vi "Parse.vi"(8 "Error In":errorcluster, 11 "object in":refnum<class "2024_13.lvclass">) -> (0 "Error Out":errorcluster, 3 "object out":refnum<class "2024_13.lvclass">)   [LabVIEW 2023, in "2024_13.lvclass"]
uses:
  2024_13.lvclass
  Game.ctl
  Common/AOC_XY.ctl
  2024_13.lvclass/2024_13.ctl
  <vilib>/Utility/error.llb/Trim Whitespace One-Sided.vi
  <userlib>/_OpenG.lib/string/string.llb/openg_string.lvlib
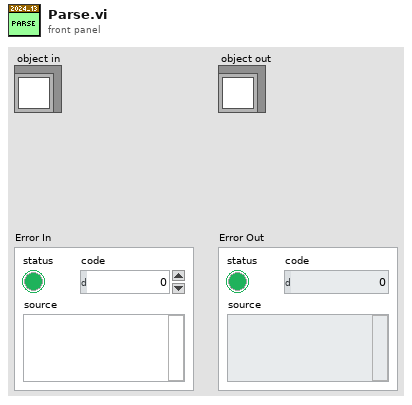
[diagram p1: front panel]
types:
  T1 = typedef "2024_13.lvclass/Game.ctl" = cluster{"A":T2, "B":T2, "Prize":T2}
  T2 = typedef "AOC_XY.ctl" = cluster{"X":u64, "Y":u64}
diagram:
  (unwired) "Button A: X+94, Y+34\nButton B: X+22, Y+67\nPrize: X=8400, Y=5400\n\nButton A: X+26, Y+66\nButton B: X+67, Y+21\nPrize: X=12748, Y=12176\n\nButton A: X+17, Y+86\nButton B: X+84, Y+37\nPrize: X=7870, Y=6450\n\nButton A: X+69, Y+23\nButton B: X+27, Y+71\nPrize: X=18641, Y=10279" ("PuzzleInput")
  n1 = call <vilib>:"Trim Whitespace.vi"("string"="Button A: X+97, Y+12\nButton B: X+52, Y+63\nPrize: X=10471, Y=4350\n\nButton A: X+79, Y+41\nButton B: X+29, Y+68\nPrize: X=7216, Y=8987\n\nButton A: X+13, Y+68\nButton B: X+46, Y+16\nPrize: X=1226, Y=8336\n\nButton A: X+14, Y+42\nButton B: X+63, Y+23\nPrize: X=15649, Y=1769\n\nButton A: X+59, Y+19\nButton B: X+53, Y+95\nPrize: X=8976, Y=10450\n\nButton A: X+91, Y+84\nButton B: X+19, Y+92\nPrize: X=9023, Y=13020\n\nButton A: X+14, Y+33\nButton B: X+26, Y+12\nPrize: X=4032, Y=8054\n\nButton A: X+69, Y+83\nButton B: X+70, Y+18\nPrize: X=8868, Y=8284\n\nButton A: X+14, Y+47\nButton B: X+83, Y+51\nPrize: X=7081, Y=7154\n\nButton A: X+33, Y+67\nButton B: X+50, Y+17\nPrize: X=12916, Y=4279\n\nButton A: X+22, Y+75\nButton B: X+77, Y+23\nPrize: X=12981, Y=9742\n\nButton A: X+90, Y+30\nButton B: X+17, Y+33\nPrize: X=6270, Y=2910\n\nButton A: X+62, Y+11\nButton B: X+43, Y+65\nPrize: X=3850, Y=1601\n\nButton A: X+48, Y+21\nButton B: X+21, Y+33\nPrize: X=8108, Y=1334\n\nButton A: X+12, Y+40\nButton B: X+49, Y+23\nPrize: X=12471, Y=11957\n\nButton A: X+86, Y+11\nButton B: X+56, Y+69\nPrize: X=4404, Y=1058\n\nButton A: X+80, Y+26\nButton B: X+11, Y+57\nPrize: X=6899, Y=5923\n\nButton A: X+25, Y+51\nButton B: X+59, Y+24\nPrize: X=14076, Y=10916\n\nButton A: X+48, Y+46\nButton B: X+13, Y+94\nPrize: X=1915, Y=6320\n\nButton A: X+47, Y+32\nButton B: X+20, Y+44\nPrize: X=19516, Y=14572\n\nButton A: X+84, Y+21\nButton B: X+13, Y+89\nPrize: X=4350, Y=2631\n\nButton A: X+29, Y+85\nButton B: X+33, Y+26\nPrize: X=4361, Y=7973\n\nButton A: X+78, Y+35\nButton B: X+11, Y+42\nPrize: X=9808, Y=10623\n\nButton A: X+35, Y+64\nButton B: X+38, Y+15\nPrize: X=4993, Y=274\n\nButton A: X+18, Y+47\nButton B: X+54, Y+15\nPrize: X=10646, Y=16999\n\nButton A: X+99, Y+55\nButton B: X+18, Y+75\nPrize: X=5256, Y=5455\n\nButton A: X+83, Y+91\nButton B: X+11, Y+58\nPrize: X=3635, Y=4261\n\nButton A: X+60, Y+27\nButton B: X+29, Y+56\nPrize: X=740, Y=11114\n\nButton A: X+59, Y+15\nButton B: X+29, Y+75\nPrize: X=14539, Y=13025\n\nButton A: X+67, Y+23\nButton B: X+11, Y+57\nPrize: X=2430, Y=2218\n\nButton A: X+80, Y+45\nButton B: X+37, Y+82\nPrize: X=9822, Y=10787\n\nButton A: X+11, Y+45\nButton B: X+51, Y+23\nPrize: X=1269, Y=18697\n\nButton A: X+56, Y+32\nButton B: X+16, Y+50\nPrize: X=9080, Y=15276\n\nButton A: X+93, Y+93\nButton B: X+11, Y+90\nPrize: X=4103, Y=11529\n\nButton A: X+24, Y+21\nButton B: X+12, Y+51\nPrize: X=2016, Y=3627\n\nButton A: X+72, Y+41\nButton B: X+25, Y+80\nPrize: X=3812, Y=3486\n\nButton A: X+29, Y+14\nButton B: X+22, Y+53\nPrize: X=2677, Y=14205\n\nButton A: X+56, Y+18\nButton B: X+19, Y+69\nPrize: X=4292, Y=8432\n\nButton A: X+64, Y+16\nButton B: X+14, Y+50\nPrize: X=3752, Y=536\n\nButton A: X+45, Y+31\nButton B: X+26, Y+59\nPrize: X=4694, Y=5247\n\nButton A: X+61, Y+21\nButton B: X+19, Y+48\nPrize: X=3931, Y=257\n\nButton A: X+13, Y+36\nButton B: X+68, Y+26\nPrize: X=17218, Y=17896\n\nButton A: X+15, Y+81\nButton B: X+31, Y+21\nPrize: X=2580, Y=7344\n\nButton A: X+78, Y+51\nButton B: X+12, Y+34\nPrize: X=3380, Y=16870\n\nButton A: X+86, Y+29\nButton B: X+52, Y+60\nPrize: X=5118, Y=2745\n\nButton A: X+12, Y+49\nButton B: X+77, Y+16\nPrize: X=7847, Y=7211\n\nButton A: X+30, Y+49\nButton B: X+48, Y+19\nPrize: X=1034, Y=15377\n\nButton A: X+25, Y+61\nButton B: X+26, Y+12\nPrize: X=6825, Y=14177\n\nButton A: X+59, Y+20\nButton B: X+11, Y+23\nPrize: X=13324, Y=946\n\nButton A: X+36, Y+54\nButton B: X+29, Y+13\nPrize: X=4435, Y=12219\n\nButton A: X+17, Y+77\nButton B: X+61, Y+17\nPrize: X=2681, Y=5661\n\nButton A: X+41, Y+19\nButton B: X+25, Y+55\nPrize: X=4484, Y=9416\n\nButton A: X+26, Y+68\nButton B: X+70, Y+26\nPrize: X=8284, Y=10434\n\nButton A: X+54, Y+11\nButton B: X+25, Y+78\nPrize: X=11040, Y=7758\n\nButton A: X+85, Y+23\nButton B: X+54, Y+74\nPrize: X=2400, Y=2728\n\nButton A: X+93, Y+29\nButton B: X+13, Y+22\nPrize: X=7293, Y=2328\n\nButton A: X+23, Y+87\nButton B: X+48, Y+20\nPrize: X=2279, Y=4743\n\nButton A: X+83, Y+34\nButton B: X+32, Y+43\nPrize: X=7734, Y=4035\n\nButton A: X+25, Y+61\nButton B: X+83, Y+44\nPrize: X=6884, Y=5225\n\nButton A: X+27, Y+58\nButton B: X+98, Y+47\nPrize: X=7921, Y=3934\n\nButton A: X+31, Y+57\nButton B: X+33, Y+14\nPrize: X=3052, Y=3838\n\nButton A: X+96, Y+18\nButton B: X+77, Y+97\nPrize: X=6503, Y=6751\n\nButton A: X+11, Y+29\nButton B: X+71, Y+36\nPrize: X=1000, Y=671\n\nButton A: X+25, Y+53\nButton B: X+44, Y+20\nPrize: X=13129, Y=17325\n\nButton A: X+33, Y+13\nButton B: X+50, Y+66\nPrize: X=3194, Y=9314\n\nButton A: X+54, Y+15\nButton B: X+24, Y+64\nPrize: X=19418, Y=8601\n\nButton A: X+13, Y+46\nButton B: X+56, Y+14\nPrize: X=10671, Y=11208\n\nButton A: X+35, Y+91\nButton B: X+25, Y+14\nPrize: X=2700, Y=6153\n\nButton A: X+85, Y+25\nButton B: X+16, Y+97\nPrize: X=2407, Y=1354\n\nButton A: X+24, Y+12\nButton B: X+13, Y+30\nPrize: X=3299, Y=3318\n\nButton A: X+17, Y+46\nButton B: X+50, Y+24\nPrize: X=17242, Y=6760\n\nButton A: X+20, Y+43\nButton B: X+26, Y+14\nPrize: X=2474, Y=748\n\nButton A: X+19, Y+78\nButton B: X+90, Y+12\nPrize: X=9966, Y=7668\n\nButton A: X+96, Y+77\nButton B: X+26, Y+73\nPrize: X=3708, Y=5790\n\nButton A: X+37, Y+77\nButton B: X+51, Y+15\nPrize: X=13364, Y=12440\n\nButton A: X+30, Y+78\nButton B: X+76, Y+31\nPrize: X=6378, Y=3588\n\nButton A: X+60, Y+26\nButton B: X+13, Y+25\nPrize: X=10780, Y=7426\n\nButton A: X+33, Y+40\nButton B: X+59, Y+16\nPrize: X=4212, Y=3440\n\nButton A: X+30, Y+11\nButton B: X+25, Y+40\nPrize: X=1145, Y=1499\n\nButton A: X+14, Y+30\nButton B: X+48, Y+15\nPrize: X=4416, Y=3840\n\nButton A: X+45, Y+68\nButton B: X+59, Y+25\nPrize: X=6633, Y=5404\n\nButton A: X+34, Y+62\nButton B: X+44, Y+19\nPrize: X=9234, Y=16930\n\nButton A: X+65, Y+12\nButton B: X+16, Y+42\nPrize: X=13586, Y=10016\n\nButton A: X+16, Y+86\nButton B: X+63, Y+54\nPrize: X=2515, Y=5264\n\nButton A: X+40, Y+88\nButton B: X+91, Y+56\nPrize: X=3728, Y=7048\n\nButton A: X+43, Y+79\nButton B: X+91, Y+30\nPrize: X=5407, Y=1977\n\nButton A: X+87, Y+16\nButton B: X+86, Y+76\nPrize: X=3366, Y=2244\n\nButton A: X+39, Y+74\nButton B: X+94, Y+32\nPrize: X=6130, Y=6216\n\nButton A: X+91, Y+50\nButton B: X+24, Y+71\nPrize: X=9174, Y=7411\n\nButton A: X+81, Y+55\nButton B: X+14, Y+95\nPrize: X=4359, Y=7320\n\nButton A: X+26, Y+78\nButton B: X+79, Y+58\nPrize: X=8792, Y=11698\n\nButton A: X+81, Y+58\nButton B: X+21, Y+70\nPrize: X=8145, Y=9130\n\nButton A: X+29, Y+60\nButton B: X+83, Y+29\nPrize: X=9583, Y=6839\n\nButton A: X+72, Y+27\nButton B: X+23, Y+63\nPrize: X=16485, Y=8540\n\nButton A: X+18, Y+30\nButton B: X+47, Y+13\nPrize: X=3031, Y=8157\n\nButton A: X+36, Y+14\nButton B: X+52, Y+70\nPrize: X=19584, Y=5184\n\nButton A: X+13, Y+36\nButton B: X+32, Y+23\nPrize: X=12901, Y=6580\n\nButton A: X+34, Y+66\nButton B: X+57, Y+24\nPrize: X=13320, Y=4832\n\nButton A: X+79, Y+26\nButton B: X+65, Y+85\nPrize: X=7528, Y=2732\n\nButton A: X+20, Y+58\nButton B: X+96, Y+75\nPrize: X=3288, Y=5874\n\nButton A: X+89, Y+24\nButton B: X+35, Y+67\nPrize: X=3458, Y=5595\n\nButton A: X+63, Y+81\nButton B: X+67, Y+22\nPrize: X=4988, Y=3206\n\nButton A: X+17, Y+55\nButton B: X+54, Y+13\nPrize: X=17532, Y=19258\n\nButton A: X+30, Y+94\nButton B: X+93, Y+32\nPrize: X=2874, Y=4336\n\nButton A: X+31, Y+17\nButton B: X+24, Y+40\nPrize: X=2311, Y=8105\n\nButton A: X+58, Y+27\nButton B: X+19, Y+60\nPrize: X=6022, Y=6398\n\nButton A: X+13, Y+67\nButton B: X+84, Y+29\nPrize: X=2843, Y=2323\n\nButton A: X+56, Y+12\nButton B: X+23, Y+81\nPrize: X=2380, Y=11120\n\nButton A: X+15, Y+65\nButton B: X+56, Y+24\nPrize: X=5230, Y=5170\n\nButton A: X+19, Y+47\nButton B: X+72, Y+34\nPrize: X=17967, Y=11841\n\nButton A: X+16, Y+41\nButton B: X+78, Y+60\nPrize: X=5144, Y=4789\n\nButton A: X+52, Y+15\nButton B: X+16, Y+65\nPrize: X=19732, Y=7355\n\nButton A: X+21, Y+81\nButton B: X+71, Y+16\nPrize: X=17221, Y=9366\n\nButton A: X+61, Y+33\nButton B: X+49, Y+87\nPrize: X=8507, Y=9381\n\nButton A: X+67, Y+21\nButton B: X+15, Y+52\nPrize: X=16737, Y=7411\n\nButton A: X+33, Y+49\nButton B: X+34, Y+11\nPrize: X=6660, Y=4300\n\nButton A: X+19, Y+81\nButton B: X+96, Y+33\nPrize: X=10734, Y=10392\n\nButton A: X+60, Y+13\nButton B: X+63, Y+65\nPrize: X=7395, Y=3913\n\nButton A: X+15, Y+21\nButton B: X+96, Y+35\nPrize: X=6417, Y=3815\n\nButton A: X+20, Y+39\nButton B: X+57, Y+27\nPrize: X=611, Y=4760\n\nButton A: X+68, Y+97\nButton B: X+87, Y+37\nPrize: X=11894, Y=9824\n\nButton A: X+13, Y+81\nButton B: X+59, Y+12\nPrize: X=18946, Y=3392\n\nButton A: X+30, Y+83\nButton B: X+57, Y+11\nPrize: X=3482, Y=19301\n\nButton A: X+94, Y+11\nButton B: X+35, Y+92\nPrize: X=11544, Y=7680\n\nButton A: X+45, Y+19\nButton B: X+30, Y+45\nPrize: X=11315, Y=17659\n\nButton A: X+25, Y+42\nButton B: X+79, Y+21\nPrize: X=7695, Y=3990\n\nButton A: X+95, Y+91\nButton B: X+55, Y+13\nPrize: X=10575, Y=9217\n\nButton A: X+27, Y+46\nButton B: X+81, Y+26\nPrize: X=5508, Y=2776\n\nButton A: X+20, Y+53\nButton B: X+29, Y+17\nPrize: X=10985, Y=16700\n\nButton A: X+55, Y+74\nButton B: X+58, Y+20\nPrize: X=8888, Y=8128\n\nButton A: X+40, Y+27\nButton B: X+19, Y+43\nPrize: X=5535, Y=1095\n\nButton A: X+19, Y+72\nButton B: X+54, Y+22\nPrize: X=3261, Y=2678\n\nButton A: X+79, Y+39\nButton B: X+38, Y+75\nPrize: X=7120, Y=6102\n\nButton A: X+26, Y+91\nButton B: X+99, Y+25\nPrize: X=1223, Y=2673\n\nButton A: X+15, Y+28\nButton B: X+58, Y+23\nPrize: X=1519, Y=5600\n\nButton A: X+18, Y+53\nButton B: X+71, Y+27\nPrize: X=11055, Y=3487\n\nButton A: X+14, Y+50\nButton B: X+52, Y+18\nPrize: X=3908, Y=8576\n\nButton A: X+38, Y+17\nButton B: X+23, Y+50\nPrize: X=7788, Y=8394\n\nButton A: X+72, Y+20\nButton B: X+19, Y+68\nPrize: X=10586, Y=4272\n\nButton A: X+28, Y+66\nButton B: X+62, Y+12\nPrize: X=19418, Y=7934\n\nButton A: X+11, Y+20\nButton B: X+49, Y+24\nPrize: X=2957, Y=2252\n\nButton A: X+60, Y+11\nButton B: X+27, Y+84\nPrize: X=3146, Y=1936\n\nButton A: X+18, Y+11\nButton B: X+11, Y+41\nPrize: X=9360, Y=18112\n\nButton A: X+70, Y+31\nButton B: X+15, Y+62\nPrize: X=13135, Y=7958\n\nButton A: X+74, Y+35\nButton B: X+11, Y+41\nPrize: X=19668, Y=14478\n\nButton A: X+53, Y+89\nButton B: X+54, Y+23\nPrize: X=9521, Y=10100\n\nButton A: X+13, Y+61\nButton B: X+68, Y+28\nPrize: X=11028, Y=12380\n\nButton A: X+42, Y+29\nButton B: X+20, Y+74\nPrize: X=1906, Y=1617\n\nButton A: X+44, Y+13\nButton B: X+23, Y+60\nPrize: X=13690, Y=9554\n\nButton A: X+54, Y+16\nButton B: X+11, Y+23\nPrize: X=3792, Y=4614\n\nButton A: X+28, Y+11\nButton B: X+34, Y+63\nPrize: X=13092, Y=15599\n\nButton A: X+61, Y+14\nButton B: X+33, Y+73\nPrize: X=18520, Y=772\n\nButton A: X+64, Y+29\nButton B: X+14, Y+78\nPrize: X=3988, Y=4530\n\nButton A: X+18, Y+45\nButton B: X+54, Y+26\nPrize: X=18170, Y=10118\n\nButton A: X+70, Y+26\nButton B: X+11, Y+43\nPrize: X=6905, Y=329\n\nButton A: X+72, Y+17\nButton B: X+27, Y+58\nPrize: X=7461, Y=6253\n\nButton A: X+57, Y+45\nButton B: X+18, Y+85\nPrize: X=2340, Y=5670\n\nButton A: X+17, Y+81\nButton B: X+47, Y+35\nPrize: X=5532, Y=8220\n\nButton A: X+14, Y+60\nButton B: X+78, Y+22\nPrize: X=10172, Y=5672\n\nButton A: X+62, Y+13\nButton B: X+17, Y+65\nPrize: X=7711, Y=8089\n\nButton A: X+22, Y+38\nButton B: X+40, Y+21\nPrize: X=15254, Y=15785\n\nButton A: X+83, Y+39\nButton B: X+32, Y+71\nPrize: X=2416, Y=3038\n\nButton A: X+29, Y+62\nButton B: X+68, Y+18\nPrize: X=6454, Y=3990\n\nButton A: X+15, Y+38\nButton B: X+72, Y+33\nPrize: X=3575, Y=8334\n\nButton A: X+81, Y+15\nButton B: X+13, Y+83\nPrize: X=11268, Y=10108\n\nButton A: X+67, Y+17\nButton B: X+12, Y+76\nPrize: X=11957, Y=5399\n\nButton A: X+13, Y+97\nButton B: X+44, Y+54\nPrize: X=2788, Y=7636\n\nButton A: X+14, Y+47\nButton B: X+68, Y+30\nPrize: X=2678, Y=9911\n\nButton A: X+75, Y+16\nButton B: X+22, Y+26\nPrize: X=1049, Y=586\n\nButton A: X+16, Y+77\nButton B: X+38, Y+25\nPrize: X=2368, Y=7607\n\nButton A: X+75, Y+91\nButton B: X+77, Y+20\nPrize: X=4076, Y=3991\n\nButton A: X+64, Y+19\nButton B: X+35, Y+74\nPrize: X=8653, Y=7594\n\nButton A: X+33, Y+81\nButton B: X+57, Y+15\nPrize: X=10661, Y=2849\n\nButton A: X+11, Y+52\nButton B: X+70, Y+22\nPrize: X=1390, Y=2864\n\nButton A: X+21, Y+40\nButton B: X+21, Y+13\nPrize: X=5954, Y=5203\n\nButton A: X+52, Y+21\nButton B: X+13, Y+64\nPrize: X=11131, Y=9958\n\nButton A: X+11, Y+42\nButton B: X+95, Y+52\nPrize: X=1604, Y=4260\n\nButton A: X+63, Y+13\nButton B: X+22, Y+82\nPrize: X=670, Y=17610\n\nButton A: X+16, Y+88\nButton B: X+84, Y+74\nPrize: X=3184, Y=6648\n\nButton A: X+77, Y+14\nButton B: X+92, Y+88\nPrize: X=13208, Y=8816\n\nButton A: X+63, Y+67\nButton B: X+82, Y+13\nPrize: X=8310, Y=3940\n\nButton A: X+57, Y+16\nButton B: X+17, Y+48\nPrize: X=10242, Y=5248\n\nButton A: X+17, Y+72\nButton B: X+36, Y+37\nPrize: X=3710, Y=5667\n\nButton A: X+69, Y+22\nButton B: X+29, Y+54\nPrize: X=5207, Y=5330\n\nButton A: X+23, Y+82\nButton B: X+49, Y+11\nPrize: X=2320, Y=2070\n\nButton A: X+66, Y+27\nButton B: X+16, Y+45\nPrize: X=11344, Y=9314\n\nButton A: X+56, Y+12\nButton B: X+23, Y+66\nPrize: X=13879, Y=14258\n\nButton A: X+60, Y+22\nButton B: X+18, Y+91\nPrize: X=1668, Y=4494\n\nButton A: X+33, Y+11\nButton B: X+31, Y+68\nPrize: X=6069, Y=13315\n\nButton A: X+14, Y+37\nButton B: X+59, Y+14\nPrize: X=2210, Y=5344\n\nButton A: X+80, Y+18\nButton B: X+33, Y+94\nPrize: X=4128, Y=9240\n\nButton A: X+40, Y+17\nButton B: X+28, Y+45\nPrize: X=3436, Y=3526\n\nButton A: X+16, Y+53\nButton B: X+50, Y+22\nPrize: X=642, Y=18961\n\nButton A: X+17, Y+39\nButton B: X+65, Y+23\nPrize: X=9566, Y=11794\n\nButton A: X+66, Y+35\nButton B: X+30, Y+76\nPrize: X=8010, Y=8394\n\nButton A: X+52, Y+75\nButton B: X+37, Y+15\nPrize: X=335, Y=19220\n\nButton A: X+36, Y+29\nButton B: X+30, Y+89\nPrize: X=3690, Y=4334\n\nButton A: X+31, Y+58\nButton B: X+50, Y+20\nPrize: X=8178, Y=17844\n\nButton A: X+82, Y+22\nButton B: X+89, Y+90\nPrize: X=4306, Y=1552\n\nButton A: X+12, Y+42\nButton B: X+99, Y+75\nPrize: X=1173, Y=3291\n\nButton A: X+23, Y+57\nButton B: X+40, Y+19\nPrize: X=2246, Y=9772\n\nButton A: X+18, Y+42\nButton B: X+95, Y+15\nPrize: X=9610, Y=4650\n\nButton A: X+20, Y+57\nButton B: X+59, Y+21\nPrize: X=10072, Y=16868\n\nButton A: X+23, Y+34\nButton B: X+42, Y+15\nPrize: X=6683, Y=16946\n\nButton A: X+55, Y+73\nButton B: X+30, Y+11\nPrize: X=4150, Y=3001\n\nButton A: X+22, Y+82\nButton B: X+73, Y+12\nPrize: X=16713, Y=15870\n\nButton A: X+14, Y+53\nButton B: X+65, Y+35\nPrize: X=3017, Y=4034\n\nButton A: X+25, Y+53\nButton B: X+46, Y+19\nPrize: X=13804, Y=8575\n\nButton A: X+29, Y+13\nButton B: X+38, Y+60\nPrize: X=14048, Y=11678\n\nButton A: X+57, Y+21\nButton B: X+61, Y+83\nPrize: X=6297, Y=7041\n\nButton A: X+18, Y+99\nButton B: X+77, Y+75\nPrize: X=2549, Y=3216\n\nButton A: X+59, Y+22\nButton B: X+17, Y+33\nPrize: X=11044, Y=13465\n\nButton A: X+40, Y+17\nButton B: X+47, Y+77\nPrize: X=17101, Y=14482\n\nButton A: X+34, Y+14\nButton B: X+20, Y+38\nPrize: X=594, Y=572\n\nButton A: X+26, Y+62\nButton B: X+35, Y+11\nPrize: X=6771, Y=8811\n\nButton A: X+20, Y+33\nButton B: X+93, Y+21\nPrize: X=5259, Y=2982\n\nButton A: X+89, Y+60\nButton B: X+13, Y+91\nPrize: X=9182, Y=14167\n\nButton A: X+28, Y+98\nButton B: X+98, Y+63\nPrize: X=5712, Y=8792\n\nButton A: X+67, Y+94\nButton B: X+39, Y+15\nPrize: X=7520, Y=7532\n\nButton A: X+38, Y+17\nButton B: X+25, Y+38\nPrize: X=19009, Y=14132\n\nButton A: X+18, Y+51\nButton B: X+85, Y+39\nPrize: X=9247, Y=7833\n\nButton A: X+40, Y+92\nButton B: X+55, Y+23\nPrize: X=2390, Y=1978\n\nButton A: X+63, Y+39\nButton B: X+24, Y+51\nPrize: X=7448, Y=17612\n\nButton A: X+95, Y+25\nButton B: X+33, Y+64\nPrize: X=11557, Y=8241\n\nButton A: X+40, Y+23\nButton B: X+21, Y+73\nPrize: X=3186, Y=5853\n\nButton A: X+89, Y+81\nButton B: X+13, Y+91\nPrize: X=5270, Y=6538\n\nButton A: X+69, Y+17\nButton B: X+21, Y+64\nPrize: X=10955, Y=8181\n\nButton A: X+59, Y+15\nButton B: X+21, Y+77\nPrize: X=6203, Y=4791\n\nButton A: X+25, Y+45\nButton B: X+36, Y+21\nPrize: X=12604, Y=18854\n\nButton A: X+67, Y+17\nButton B: X+21, Y+70\nPrize: X=7506, Y=17163\n\nButton A: X+78, Y+53\nButton B: X+27, Y+89\nPrize: X=2391, Y=7065\n\nButton A: X+68, Y+26\nButton B: X+23, Y+62\nPrize: X=13179, Y=7794\n\nButton A: X+18, Y+44\nButton B: X+54, Y+16\nPrize: X=18710, Y=4780\n\nButton A: X+16, Y+36\nButton B: X+69, Y+48\nPrize: X=6028, Y=5412\n\nButton A: X+45, Y+24\nButton B: X+34, Y+73\nPrize: X=4185, Y=4701\n\nButton A: X+12, Y+26\nButton B: X+64, Y+29\nPrize: X=8628, Y=3714\n\nButton A: X+53, Y+16\nButton B: X+26, Y+65\nPrize: X=15387, Y=3502\n\nButton A: X+48, Y+17\nButton B: X+49, Y+80\nPrize: X=19364, Y=6034\n\nButton A: X+34, Y+70\nButton B: X+45, Y+21\nPrize: X=3861, Y=2289\n\nButton A: X+39, Y+76\nButton B: X+80, Y+14\nPrize: X=8169, Y=3574\n\nButton A: X+79, Y+35\nButton B: X+45, Y+74\nPrize: X=7247, Y=6887\n\nButton A: X+33, Y+19\nButton B: X+12, Y+49\nPrize: X=7163, Y=16959\n\nButton A: X+24, Y+11\nButton B: X+30, Y+49\nPrize: X=11852, Y=4499\n\nButton A: X+32, Y+11\nButton B: X+25, Y+70\nPrize: X=5331, Y=15303\n\nButton A: X+98, Y+63\nButton B: X+18, Y+68\nPrize: X=5564, Y=5044\n\nButton A: X+85, Y+11\nButton B: X+41, Y+76\nPrize: X=10558, Y=6527\n\nButton A: X+20, Y+48\nButton B: X+45, Y+11\nPrize: X=10755, Y=17297\n\nButton A: X+37, Y+23\nButton B: X+23, Y+51\nPrize: X=12782, Y=14840\n\nButton A: X+37, Y+69\nButton B: X+44, Y+11\nPrize: X=4057, Y=15396\n\nButton A: X+21, Y+43\nButton B: X+55, Y+30\nPrize: X=6148, Y=18269\n\nButton A: X+32, Y+63\nButton B: X+32, Y+17\nPrize: X=8032, Y=16179\n\nButton A: X+81, Y+68\nButton B: X+18, Y+51\nPrize: X=3429, Y=6001\n\nButton A: X+90, Y+27\nButton B: X+36, Y+96\nPrize: X=8910, Y=3099\n\nButton A: X+68, Y+36\nButton B: X+18, Y+44\nPrize: X=494, Y=6740\n\nButton A: X+65, Y+11\nButton B: X+13, Y+71\nPrize: X=809, Y=7803\n\nButton A: X+29, Y+40\nButton B: X+97, Y+24\nPrize: X=10076, Y=3248\n\nButton A: X+83, Y+33\nButton B: X+17, Y+81\nPrize: X=5639, Y=4395\n\nButton A: X+22, Y+33\nButton B: X+47, Y+22\nPrize: X=7651, Y=1299\n\nButton A: X+58, Y+25\nButton B: X+16, Y+31\nPrize: X=10590, Y=3747\n\nButton A: X+36, Y+14\nButton B: X+36, Y+71\nPrize: X=7856, Y=1885\n\nButton A: X+64, Y+18\nButton B: X+74, Y+89\nPrize: X=9164, Y=5714\n\nButton A: X+82, Y+51\nButton B: X+22, Y+99\nPrize: X=7542, Y=10407\n\nButton A: X+43, Y+18\nButton B: X+34, Y+65\nPrize: X=17803, Y=6032\n\nButton A: X+62, Y+39\nButton B: X+19, Y+44\nPrize: X=15584, Y=11902\n\nButton A: X+32, Y+24\nButton B: X+33, Y+83\nPrize: X=2199, Y=4853\n\nButton A: X+14, Y+60\nButton B: X+80, Y+18\nPrize: X=1010, Y=6134\n\nButton A: X+71, Y+24\nButton B: X+18, Y+62\nPrize: X=3079, Y=5296\n\nButton A: X+17, Y+54\nButton B: X+53, Y+12\nPrize: X=11314, Y=7550\n\nButton A: X+42, Y+20\nButton B: X+13, Y+41\nPrize: X=7760, Y=9208\n\nButton A: X+26, Y+48\nButton B: X+46, Y+25\nPrize: X=16412, Y=3732\n\nButton A: X+20, Y+64\nButton B: X+65, Y+21\nPrize: X=6165, Y=11225\n\nButton A: X+14, Y+58\nButton B: X+68, Y+27\nPrize: X=7972, Y=15348\n\nButton A: X+46, Y+17\nButton B: X+29, Y+96\nPrize: X=3598, Y=8664\n\nButton A: X+93, Y+32\nButton B: X+28, Y+76\nPrize: X=11382, Y=9292\n\nButton A: X+65, Y+24\nButton B: X+11, Y+35\nPrize: X=2252, Y=10494\n\nButton A: X+28, Y+61\nButton B: X+46, Y+16\nPrize: X=14138, Y=7874\n\nButton A: X+49, Y+28\nButton B: X+29, Y+66\nPrize: X=2640, Y=4672\n\nButton A: X+14, Y+99\nButton B: X+98, Y+68\nPrize: X=2730, Y=5555\n\nButton A: X+54, Y+54\nButton B: X+89, Y+22\nPrize: X=5618, Y=3340\n\nButton A: X+18, Y+46\nButton B: X+76, Y+48\nPrize: X=5930, Y=2346\n\nButton A: X+78, Y+75\nButton B: X+87, Y+21\nPrize: X=3906, Y=2628\n\nButton A: X+14, Y+22\nButton B: X+41, Y+19\nPrize: X=3378, Y=12850\n\nButton A: X+69, Y+18\nButton B: X+18, Y+73\nPrize: X=6411, Y=2697\n\nButton A: X+33, Y+78\nButton B: X+70, Y+37\nPrize: X=3122, Y=6737\n\nButton A: X+14, Y+74\nButton B: X+86, Y+20\nPrize: X=6300, Y=2880\n\nButton A: X+11, Y+28\nButton B: X+48, Y+11\nPrize: X=6804, Y=16815\n\nButton A: X+62, Y+17\nButton B: X+31, Y+65\nPrize: X=6448, Y=4141\n\nButton A: X+70, Y+11\nButton B: X+72, Y+59\nPrize: X=4918, Y=1202\n\nButton A: X+97, Y+67\nButton B: X+13, Y+33\nPrize: X=8935, Y=7805\n\nButton A: X+34, Y+78\nButton B: X+76, Y+49\nPrize: X=8860, Y=10423\n\nButton A: X+27, Y+69\nButton B: X+37, Y+21\nPrize: X=1124, Y=960\n\nButton A: X+25, Y+11\nButton B: X+15, Y+53\nPrize: X=11185, Y=17987\n\nButton A: X+12, Y+57\nButton B: X+67, Y+20\nPrize: X=10831, Y=11898\n\nButton A: X+21, Y+52\nButton B: X+68, Y+37\nPrize: X=488, Y=19181\n\nButton A: X+27, Y+12\nButton B: X+30, Y+67\nPrize: X=4040, Y=8930\n\nButton A: X+84, Y+30\nButton B: X+58, Y+99\nPrize: X=4462, Y=6369\n\nButton A: X+32, Y+59\nButton B: X+37, Y+20\nPrize: X=12149, Y=3281\n\nButton A: X+44, Y+12\nButton B: X+86, Y+94\nPrize: X=7916, Y=8508\n\nButton A: X+11, Y+42\nButton B: X+64, Y+29\nPrize: X=1438, Y=7055\n\nButton A: X+13, Y+58\nButton B: X+71, Y+30\nPrize: X=1136, Y=7488\n\nButton A: X+29, Y+32\nButton B: X+15, Y+73\nPrize: X=466, Y=740\n\nButton A: X+18, Y+40\nButton B: X+60, Y+14\nPrize: X=3758, Y=16800\n\nButton A: X+29, Y+48\nButton B: X+46, Y+11\nPrize: X=823, Y=4172\n\nButton A: X+12, Y+36\nButton B: X+84, Y+21\nPrize: X=2916, Y=1818\n\nButton A: X+57, Y+98\nButton B: X+99, Y+38\nPrize: X=11955, Y=7862\n\nButton A: X+11, Y+59\nButton B: X+54, Y+19\nPrize: X=5556, Y=8121\n\nButton A: X+42, Y+16\nButton B: X+25, Y+46\nPrize: X=6595, Y=7886\n\nButton A: X+18, Y+38\nButton B: X+51, Y+33\nPrize: X=10826, Y=15950\n\nButton A: X+30, Y+52\nButton B: X+24, Y+11\nPrize: X=18374, Y=18262\n\nButton A: X+43, Y+17\nButton B: X+20, Y+51\nPrize: X=6909, Y=5174\n\nButton A: X+12, Y+49\nButton B: X+73, Y+35\nPrize: X=19520, Y=7473\n\nButton A: X+26, Y+54\nButton B: X+81, Y+18\nPrize: X=2771, Y=1098\n\nButton A: X+38, Y+16\nButton B: X+35, Y+56\nPrize: X=9775, Y=16248\n\nButton A: X+74, Y+12\nButton B: X+13, Y+83\nPrize: X=17184, Y=8706\n\nButton A: X+47, Y+15\nButton B: X+59, Y+68\nPrize: X=6455, Y=5207\n\nButton A: X+51, Y+75\nButton B: X+73, Y+35\nPrize: X=3535, Y=4475\n\nButton A: X+11, Y+49\nButton B: X+43, Y+19\nPrize: X=15272, Y=2282\n\nButton A: X+64, Y+12\nButton B: X+12, Y+73\nPrize: X=2236, Y=7049\n\nButton A: X+80, Y+36\nButton B: X+18, Y+61\nPrize: X=19208, Y=11960\n\nButton A: X+52, Y+21\nButton B: X+11, Y+35\nPrize: X=4204, Y=354\n" ("PuzzleInput")) -> ("trimmed string"=w9:string)  [unwired: 1 in]
  n2 = call <userlib>:"Multi-line String to Array__ogtk.vi"("string"=w9) -> ("lines"=w8:string[])
  n3 = Build Array (concatenate)(w8, "\n") -> (w6:string[])
  n4 = Decimate 1D Array(w6) -> (w5:string[], w4:string[], w3:string[])  [unwired: 1 out]
  n5 = for {
    tunnel: w5 -> [w34] mode=indexing
    tunnel: w4 -> [w28] mode=indexing
    tunnel: w3 -> [w18] mode=indexing
    tunnel: [w35] -> w2 mode=indexing
    w20 = u64 0 ("default value 1")
    w21 = u64 0 ("default value 1")
    w22 = u64 0 ("default value 1")
    n6 = Scan From String(format string="Button A: X+%d, Y+%d", input string=w34, default 1=w22, default 2=w22) -> (remaining string=w30:string, output 1=w32:u64, output 2=w31:u64)  [unwired: 2 in, 2 out]
    n7 = Scan From String(format string="Button B: X+%d, Y+%d", input string=w28, default 1=w21, default 2=w21) -> (remaining string=w26:string, output 1=w24:u64, output 2=w23:u64)  [unwired: 2 in, 2 out]
    n8 = Scan From String(format string="Prize: X=%d, Y=%d", input string=w18, default 1=w20, default 2=w20) -> (remaining string=w15:string, output 1=w17:u64, output 2=w16:u64)  [unwired: 2 in, 2 out]
    n9 = Bundle By Name(cluster=T1 {"A"={"X"=0, "Y"=0}, "B"={"X"=0, "Y"=0}, "Prize"={"X"=0, "Y"=0}} ("Game"), "A.X"=w32, "A.Y"=w31, "B.X"=w24, "B.Y"=w23, "Prize.X"=w17, "Prize.Y"=w16) -> (w35:T1)
    n10 = Empty String/Path?(string/path=w30) -> (empty?=w29:bool)
    n11 = Empty String/Path?(string/path=w26) -> (empty?=w25:bool)
    n12 = Empty String/Path?(string/path=w15) -> (empty?=w14:bool)
    n13 = Compound Arithmetic op=AND(w29, w25, w14) -> (w13:bool)
    n14 = case shown="False" w13 {
      frame False {
      }
      frame True {
      }
    }
  }
  n15 = Bundle By Name(cluster="object in", "Games"=w2) -> (→"object out":refnum<class "2024_13.lvclass">)
  "Error Out" <- "Error In"
